vi "Read Address.vi"(8 "error in":errorcluster, 11 "address ref in":refnum<k20>) -> (0 "error out":errorcluster, 2 "terminal":T1, 3 "address ref out":refnum<k20>)   [LabVIEW 2020, in "MIL-STD 1553 Import.lvlib"]
uses:
  MIL-STD 1553 Import.lvlib
  Shared/Terminal Endpoint.ctl
  Shared/Address.ctl
  d1480715-b761-474b-8fe5-ec7c306e7985.vi
  cef1b9ea-8129-4b98-8421-c923908517a8.vi
  e39d4d0c-c6d5-4d8d-a621-4ae47de02d87.vi
  68acfba6-3310-4a68-92ee-9cd7e900ed40.vi
  997d6892-f520-484c-a71d-f8493dde3f6b.vi/24d84408-cf52-4725-bbcd-7eb9945ef2a5.vi
  c4881378-0696-4b0e-820e-c01546609bba.vi/62a428ba-605c-405c-a8ab-4b5dc73233e9.vi
  c4881378-0696-4b0e-820e-c01546609bba.vi/5ad0f0e7-50c2-4da3-8f04-f13e20a45d4f.vi
  c4881378-0696-4b0e-820e-c01546609bba.vi/bb3dc68e-ff02-4b92-badb-778c677133f8.vi
  285a92bc-9c63-43b3-b544-62fba9bc5a66.vi/9e3e17d4-0564-4e2d-9f33-458dc60d2c00.vi
  5052c8a8-a5e7-4770-b2a7-42c35e434072.vi/b7a64bff-9641-4b34-8b47-21cad5d1d30a.vi
  5052c8a8-a5e7-4770-b2a7-42c35e434072.vi/ea477169-3e22-4d68-8fc7-2e3959d26724.vi
  5052c8a8-a5e7-4770-b2a7-42c35e434072.vi/7f19b5ef-4050-4d55-b717-c466d770bc07.vi
  997d6892-f520-484c-a71d-f8493dde3f6b.vi/b1e6fcf8-dac1-42d2-b1fe-151afe06dbd4.vi/4a4f8aea-9f6a-4abb-8f6c-edd7c0e67748.vi
  c4881378-0696-4b0e-820e-c01546609bba.vi/749400e4-5f60-4dbe-83d9-453db9d95f9d.vi/01bc7dae-9a28-448c-8f04-5cb4150716fb.vi
  c4881378-0696-4b0e-820e-c01546609bba.vi/472f3993-b042-455f-80f2-2140c22c21b8.vi/8bfb5eb3-f432-4527-8c0d-a0869d4bbd40.vi
  c4881378-0696-4b0e-820e-c01546609bba.vi/3e45ab0b-a443-4555-805a-cc6dd0adbb20.vi/f2a1435f-38ab-49e0-a290-aa9a19fc9bca.vi
  285a92bc-9c63-43b3-b544-62fba9bc5a66.vi/b1e6fcf8-dac1-42d2-b1fe-151afe06dbd4.vi/10df0ece-0d95-4b07-ab76-3a835ffe4772.vi
  5052c8a8-a5e7-4770-b2a7-42c35e434072.vi/749400e4-5f60-4dbe-83d9-453db9d95f9d.vi/15fc7374-8bd4-48cc-bd59-f87bd276733b.vi
  5052c8a8-a5e7-4770-b2a7-42c35e434072.vi/472f3993-b042-455f-80f2-2140c22c21b8.vi/69f02086-e031-47d8-bff8-5ce82ca0761f.vi
  5052c8a8-a5e7-4770-b2a7-42c35e434072.vi/3e45ab0b-a443-4555-805a-cc6dd0adbb20.vi/91f08026-48f4-4272-80f6-4b7bf9a95c63.vi
  Constants.vi
  Get Element References by Tag Name.vi
  <vilib>/xml/Get Node Text Content.vi
  <vilib>/Utility/error.llb/Error Cluster From Error Code.vi
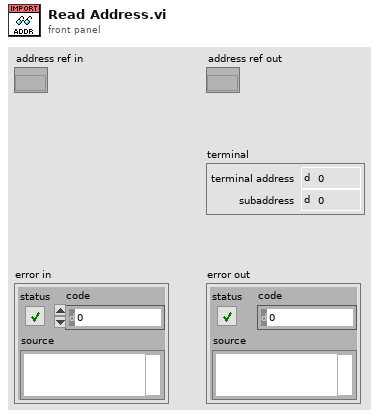
[diagram p1: front panel]
types:
  T1 = typedef "Terminal Endpoint.ctl" = cluster{"terminal address":T2, "subaddress":T2}
  T2 = typedef "Address.ctl" = u16
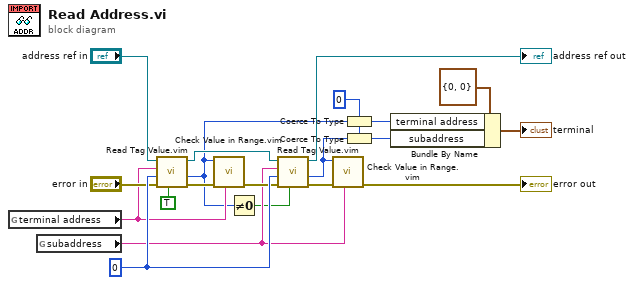
[diagram p0: block diagram]
diagram:
  w20 = u16 0 ("error code (0)")
  w17 = T2 0 ("subaddress")
  n1 = global read "Constants.vi" "terminal address"() -> (w4:string)
  n2 = global read "Constants.vi" "subaddress"() -> (w5:string)
  n3 = call "Read Tag Value.vim"("required (F)"=TRUE, "error in"="error in", "default"=w20, "tag name"=w4, "node in"="address ref in") -> ("error out"=w10:errorcluster, "value"=w2:u16, "node out"=w13:refnum<k20>)  [unwired: 4 in]
  n4 = call "Check Value in Range.vim"("element name"=w4, "error in"=w10, "value"=w2) -> ("error out"=w9:errorcluster)  [unwired: 8 in]
  n5 = Not Equal To 0?(x=w2) -> (x != 0?=w1:bool)
  n6 = call "Read Tag Value.vim"("required (F)"=w1, "error in"=w9, "default"=w20, "tag name"=w5, "node in"=w13) -> ("error out"=w8:errorcluster, "value"=w3:u16, "node out"=→"address ref out":refnum<k20>)  [unwired: 4 in]
  n7 = call "Check Value in Range.vim"("element name"=w5, "error in"=w8, "value"=w3) -> ("error out"=→"error out":errorcluster)  [unwired: 8 in]
  n8 = Coerce To Type(0:w2, 1:w17) -> (2:w15:T2)
  n9 = Coerce To Type(0:w3, 1:w17) -> (2:w16:T2)
  n10 = Bundle By Name(cluster=T1 {"terminal address"=0, "subaddress"=0} ("endpoint Rx"), "terminal address"=w15, "subaddress"=w16) -> (→"terminal":T1)
